vi "Un-Pad Start and End.vi"(0 "Padded Waveform":waveform(dbl)={"t0"=timestamp(3461330237.7970004 s since 1904-01-01), "dt"=1.0, "Y"=[9.0, 10.0, 10.5, 10.0, 8.5]}, 1 "Original Waveform":waveform(dbl)={"t0"=timestamp(3461330237.7970004 s since 1904-01-01), "dt"=1.0, "Y"=[9.0, 10.0, 10.5, 10.0, 8.5]}) -> (2 "Un-padded Waveform":waveform(dbl)={"t0"=timestamp(3461330237.7970004 s since 1904-01-01), "dt"=1.0, "Y"=[9.0, 9.0, 9.0, 9.0, 9.0, 9.0, 10.0, 10.5, 10.0, 8.5, 8.5, 8.5, 8.5, 8.5, 8.5]})   [LabVIEW 2010]
panel:
  out "XY Graph":cluster{"X array":dbl[], "Y array":dbl[]}(graph)={"X array"=[0.0, 1.0, 2.0, 3.0, 4.0, 5.0, 6.0, 7.0, 8.0, 9.0, 10.0, 11.0, 12.0, 13.0, 14.0], "Y array"=[9.0, 9.0, 9.0, 9.0, 9.0, 9.0, 10.0, 10.5, 10.0, 8.5, 8.5, 8.5, 8.5, 8.5, 8.5]}
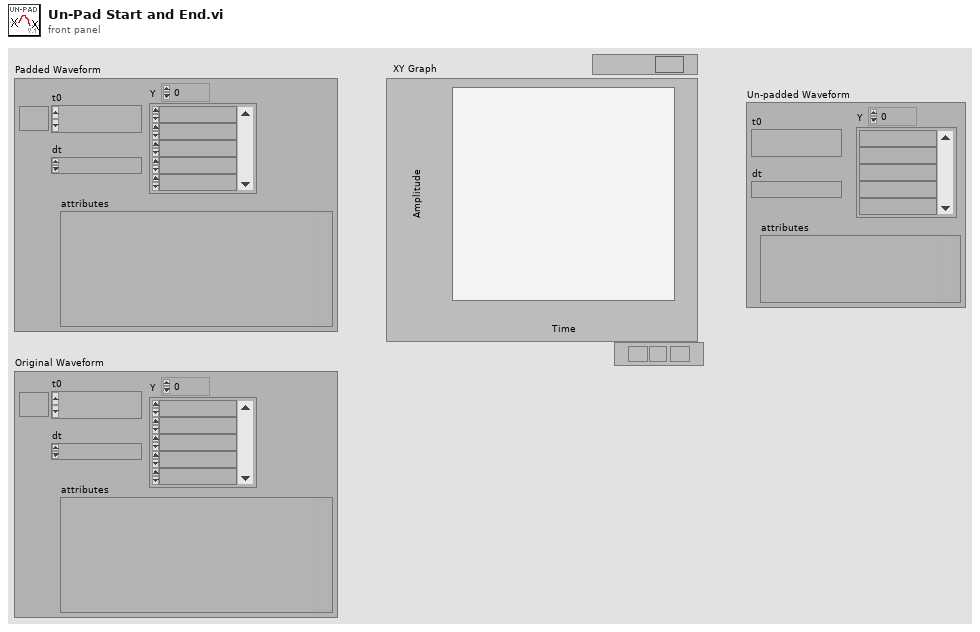
[diagram p1: front panel]
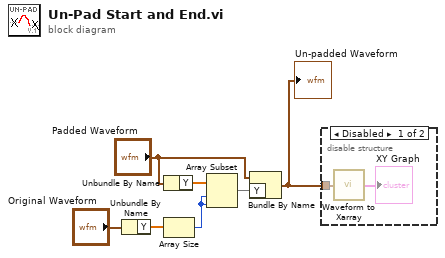
[diagram p0: block diagram]
diagram:
  n1 = Unbundle By Name("Original Waveform") -> ("Y"=w5:dbl[])
  n2 = Unbundle By Name("Padded Waveform") -> ("Y"=w2:dbl[])
  n3 = Array Size(array=w5) -> (size(s)=w3:i32)
  n4 = Array Subset(array=w2, index=w3, length=w3) -> (w1:dbl[])
  n5 = Bundle By Name(cluster="Padded Waveform", "Y"=w1) -> (w6:waveform(dbl))
  "Un-padded Waveform" <- w6
  n6 = disable-structure shown="Disabled" {
    disable-tunnel: w6 -> [w9 _]
    frame Disabled {
      n7 = call "Waveform to Xarray.vi"("Waveform In"=w9) -> ("Single Plot"=→"XY Graph":cluster{"X array":dbl[], "Y array":dbl[]})
    }
    frame Enabled {
    }
  }
